vi "Write current unit ID.vi"(8 "error in":errorcluster, 10 "request unit ID":u8, 11 "Serial Data Unit in":refnum<class "Serial Data Unit.lvclass">) -> (0 "error out":errorcluster, 3 "Serial Data Unit out":refnum<class "Serial Data Unit.lvclass">)   [LabVIEW 2021, in "Serial Data Unit.lvclass"]
uses:
  Serial Data Unit.lvclass
  Serial Data Unit.lvclass/Serial Data Unit.ctl
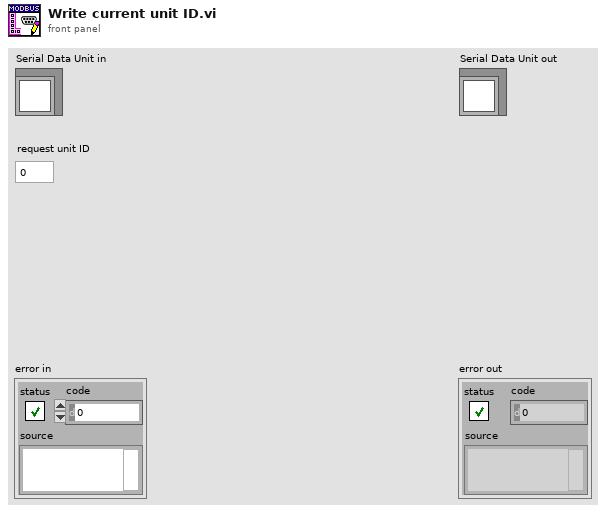
[diagram p1: front panel]
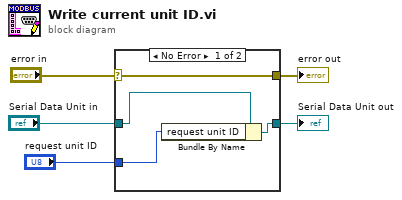
[diagram p0: block diagram]
diagram:
  n1 = case shown="No Error" "error in" {
    selector: "error in" -> [w9 w10]
    tunnel: [w9 w10] -> w4
    tunnel: [w7 w11] -> w2
    tunnel: "Serial Data Unit in" -> [w8 w11]
    tunnel: "request unit ID" -> [w6 _]
    frame No Error {
      n2 = Bundle By Name(cluster=w8, "request unit ID"=w6) -> (w7:refnum<class "Serial Data Unit.lvclass">)
    }
    frame Error {
    }
  }
  "error out" <- w4
  "Serial Data Unit out" <- w2
